vi "Controllers_PIDZPositionNoWhile.vi"(0 "Task In":refnum<k21>, 1 "SP Femto":dbl=0.1, 2 "Loop Time In":i32, 3 "Piezo In / V":dbl format="%.3g", 5 "Error In":errorcluster, 6 "Alpha":dbl=nan format="%.2f", 7 "DC Bias":dbl=0.2, 8 "Beta":dbl=1.0, 9 "PID gains":T1 {"derivative time (Td, min)" format="%.6f"; "integral time (Ti, min)" format="%.6f"; "proportional gain (Kc)" format="%.6f"}, 10 "Iterator In":i32, 11 "Real time Femto / V":dbl=0.10000000000000014, 12 "Aquisition Rate (20000) / Hz":dbl=20000.0) -> (14 "Task Out":refnum<k21>, 15 "Stop?":bool, 16 "Loop Time Out":u32, 17 "Piezo Out / V":dbl format="%.6g", 18 "Runtime / s":dbl, 19 "Error Out":errorcluster)   [LabVIEW 2025]
uses:
  <vilib>/DAQmx/write.llb/DAQmx Write (Analog 1D DBL NChan 1Samp).vi
  <vilib>/addons/control/pid/pid.llb/PID Advanced (DBL).vi
  <vilib>/DAQmx/miscellaneous.llb/DAQmx Fill In Error Info.vi
  <vilib>/addons/control/pid/NI_PID_pid.lvlib
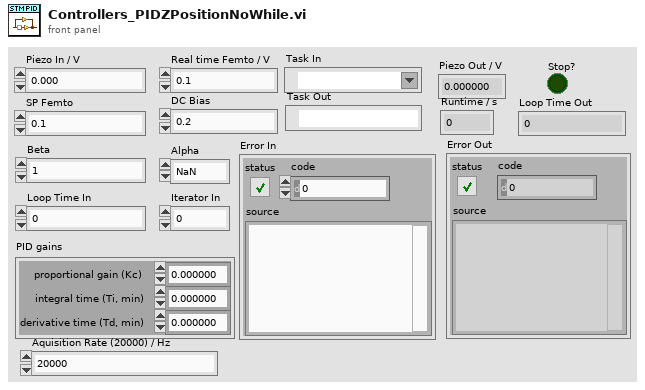
[diagram p1: front panel]
types:
  T1 = cluster{"proportional gain (Kc)":dbl, "integral time (Ti, min)":dbl, "derivative time (Td, min)":dbl}
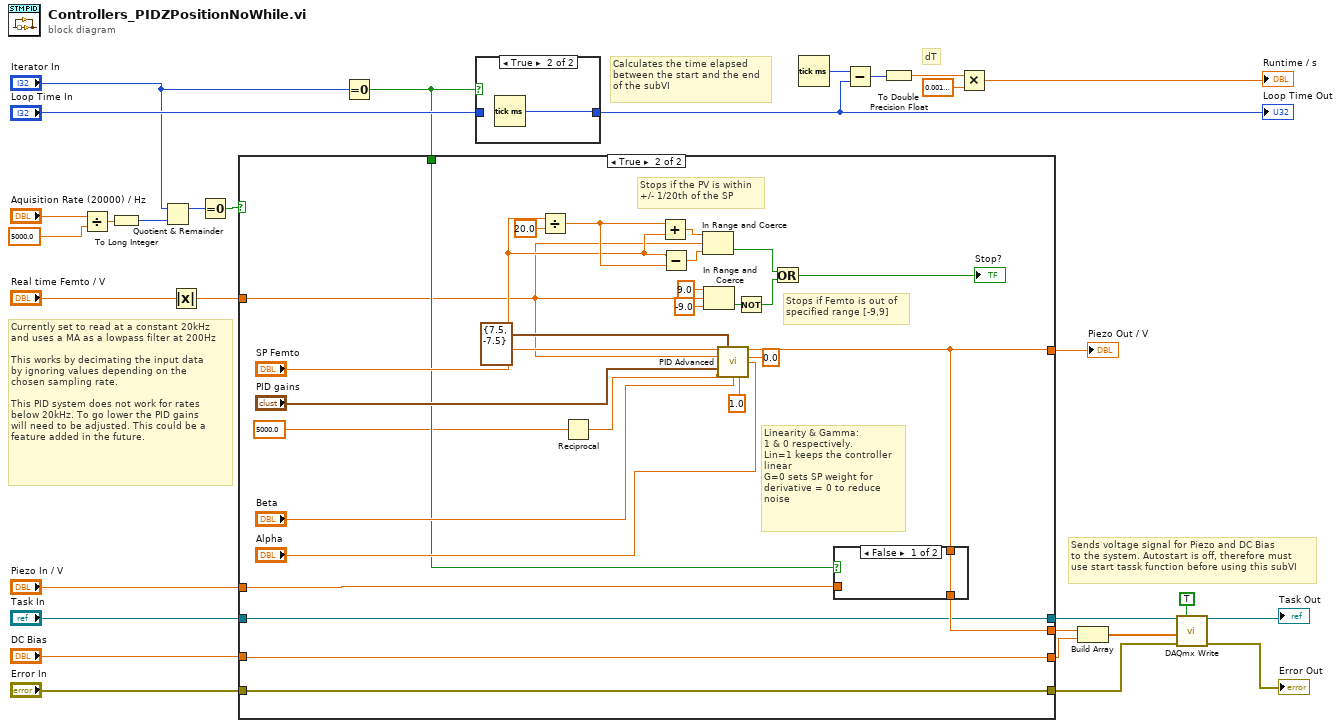
[diagram p0: block diagram]
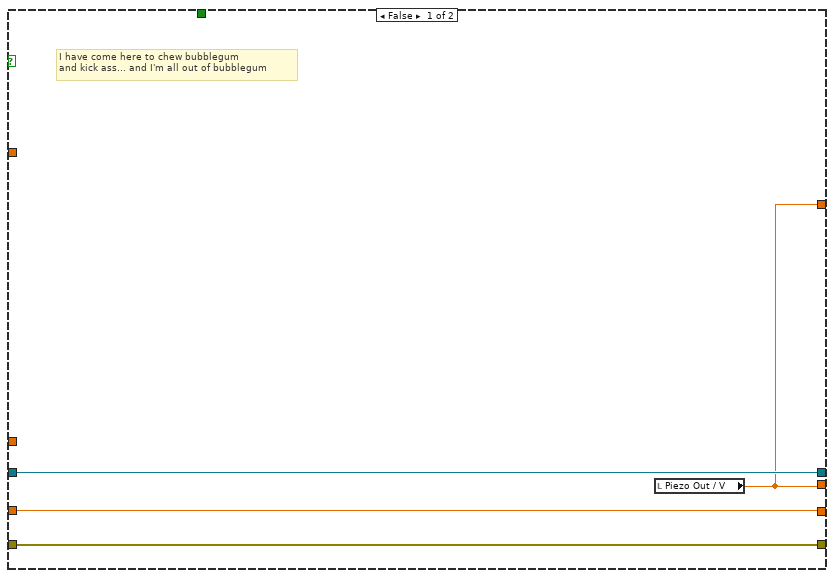
[diagram p2: hidden frame]
diagram:
  # "Currently set to read at a constant 20kHz\nand uses a MA as a lowpass filter at 200Hz\n\nThis works by decimating the input data\nby ignoring values depending on the\nchosen sampling rate. \n\nThis PID system does not work for rates\nbelow 20kHz. To go lower the PID gains\nwill need to be adjusted. This could be a\nfeature added in the future."
  # "Sends voltage signal for Piezo and DC Bias\nto the system. Autostart is off, therefore must\nuse start tassk function before using this subVI"
  # "Calculates the time elapsed\nbetween the start and the end\nof the subVI"
  # "dT"
  n1 = Divide(x="Aquisition Rate (20000) / Hz", y=5000.0) -> (x/y=w8:dbl)
  n2 = To Long Integer(number=w8) -> (32bit integer=w7:i32)
  n3 = Quotient & Remainder(x="Iterator In", y=w7) -> (x-y*floor(x/y)=w16:i32)  [unwired: 1 out]
  n4 = Absolute Value(x="Real time Femto / V") -> (abs(x)=w2:dbl)
  n5 = Equal To 0?(x=w16) -> (x = 0?=w9:bool)
  n6 = Equal To 0?(x="Iterator In") -> (x = 0?=w17:bool)
  n7 = case shown="True" w9 {
    tunnel: "Piezo In / V" -> [_ w44]
    tunnel: [w31 w42] -> w20
    tunnel: w17 -> [_ w41]
    tunnel: w2 -> [_ w36]
    tunnel: "DC Bias" -> [w33 w40]
    tunnel: [w33 w40] -> w14
    tunnel: "Error In" -> [w32 w39]
    tunnel: [w32 w39] -> w12
    tunnel: "Task In" -> [w34 w38]
    tunnel: [w34 w38] -> w10
    tunnel: [w31 w35] -> w3
    frame False {
      # "I have come here to chew bubblegum\nand kick ass... and I'm all out of bubblegum"
      n8 = local read "Piezo Out / V"() -> (w31:dbl)
    }
    frame True {
      # "Stops if Femto is out of\nspecified range [-9,9]"
      # "Linearity & Gamma:\n1 & 0 respectively.\nLin=1 keeps the controller \nlinear\nG=0 sets SP weight for \nderivative = 0 to reduce\nnoise"
      # "Stops if the PV is within\n+/- 1/20th of the SP"
      n9 = Divide(x="SP Femto", y=20.0) -> (x/y=w51:dbl)
      n10 = Reciprocal(x=5000.0) -> (1/x=w43:dbl)
      n11 = Add(x=w51, y="SP Femto") -> (x+y=w53:dbl)
      n12 = Subtract(x="SP Femto", y=w51) -> (x-y=w52:dbl)
      n13 = In Range and Coerce(upper limit=w53, x=w36, lower limit=w52) -> (In Range?=w46:bool)  [unwired: 1 out]
      n14 = In Range and Coerce(upper limit=9.0, x=w36, lower limit=-9.0) -> (In Range?=w50:bool)  [unwired: 1 out]
      n15 = call-poly <vilib>:"PID Advanced.vi"("setpoint"="SP Femto", "output range"=cluster{"output high":dbl, "output low":dbl} {"output high"=7.5, "output low"=-7.5}, "process variable"=w36, "gamma"=0.0, "alpha"="Alpha", "PID gains"="PID gains", "dt (s)"=w43, "beta"="Beta", "linearity"=1.0) -> ("output"=w35:dbl)  [unwired: 5 in, 1 out]
      n16 = Not(x=w50) -> (.not. x?=w47:bool)
      n17 = Or(x=w46, y=w47) -> (x .or. y?=→"Stop?":bool)
      n18 = case shown="False" w41 {
        tunnel: w35 -> [w62 _]
        tunnel: [w62 w63] -> w42
        tunnel: w44 -> [_ w63]
        frame False {
        }
        frame True {
        }
      }
    }
  }
  "Piezo Out / V" <- w3
  n19 = case shown="True" w17 {
    tunnel: [w64 w65] -> w29
    tunnel: "Loop Time In" -> [w64 _]
    frame False {
    }
    frame True {
      n20 = Tick Count (ms)() -> (millisecond timer value=w65:u32)
    }
  }
  "Loop Time Out" <- w29
  n21 = Tick Count (ms)() -> (millisecond timer value=w30:u32)
  n22 = Subtract(x=w30, y=w29) -> (x-y=w26:u32)
  n23 = To Double Precision Float(number=w26) -> (double precision float=w28:dbl)
  n24 = Multiply(x=w28, y=0.0010000000474974513) -> (x*y=→"Runtime / s":dbl)
  n25 = Build Array(w20, w14) -> (w19:dbl[])
  n26 = call-poly <vilib>:"DAQmx Write.vi"("task/channels in"=w10, "auto start"=TRUE, "data"=w19, "error in"=w12) -> ("task out"=→"Task Out":refnum<k21>, "error out"=→"Error Out":errorcluster)  [unwired: 9 in, 1 out]
